vi "Filter Deprecated Data.vi"(1 "Logger Parameters":T1) -> (0 "Filtered Data":dbl[][](array[numeric]))   [LabVIEW 2019, in "Telemetry Engine.lvlib"]
uses:
  Telemetry Engine.lvlib
  Types/Logger Data.ctl
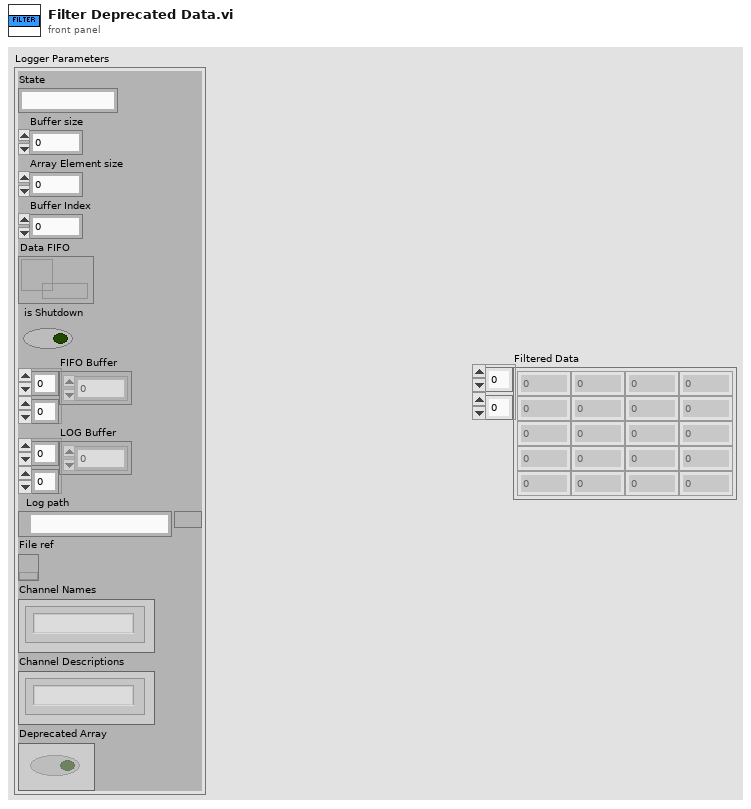
[diagram p1: front panel]
types:
  T1 = typedef "Telemetry Engine.lvlib/Logger Data.ctl" = cluster{"State":string, "Buffer size":i32, "Array Element size":i32, "Buffer Index":i32, "Data FIFO":refnum<k33>, "is Shutdown":bool, "FIFO Buffer":dbl[][], "LOG Buffer":dbl[][], "Log path":path, "File ref":refnum<k34>, "Channel Names":string[], "Channel Descriptions":string[], "Deprecated Array":bool[]}
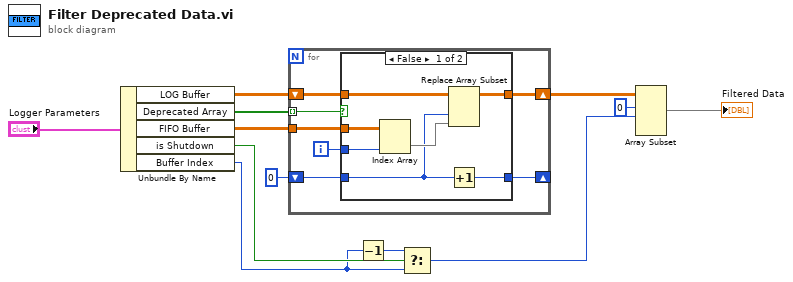
[diagram p0: block diagram]
diagram:
  n1 = Unbundle By Name("Logger Parameters") -> ("LOG Buffer"=w10:dbl[][], "Deprecated Array"=w9:bool[], "FIFO Buffer"=w8:dbl[][], "is Shutdown"=w4:bool, "Buffer Index"=w3:i32)
  n2 = for {
    tunnel: w9 -> [w13] mode=indexing
    tunnel: w8 -> [w19]
    shift-right: [w14] -> w7
    shift-left: w10 -> [w16]
    shift-right: [w15] -> _
    shift-left: 0 -> [w17]
    i -> [w18]
    n3 = case shown="False" w13 {
      tunnel: w19 -> [w26 _]
      tunnel: w18 -> [w25 _]
      tunnel: w17 -> [w22 w27]
      tunnel: w16 -> [w24 w28]
      tunnel: [w21 w27] -> w15
      tunnel: [w20 w28] -> w14
      frame False {
        n4 = Index Array(array=w26, index (col)=w25) -> (element=w23:dbl[])  [unwired: 1 in]
        n5 = Replace Array Subset(array=w24, new element=w23, index (col)=w22) -> (w20:dbl[][])  [unwired: 1 in]
        n6 = Increment(x=w22) -> (x+1=w21:i32)
      }
      frame True {
      }
    }
  }
  n7 = Decrement(x=w3) -> (x-1=w5:i32)
  n8 = Select(t=w5, s=w4, f=w3) -> (s? t:f=w2:i32)
  n9 = Array Subset(array=w7, index (row)=0 ("index"), length (row)=w2) -> (→"Filtered Data":dbl[][])  [unwired: 2 in]
